vi "Select message creator.vi"(8 "error in (no error)":errorcluster, 11 "Select control references":T2) -> (0 "error out":errorcluster, 3 "PartDetails":T1)   [LabVIEW 2019, in "ZenGage v3.0 UI.lvclass"]
uses:
  ZenGage v3.0 UI.lvclass
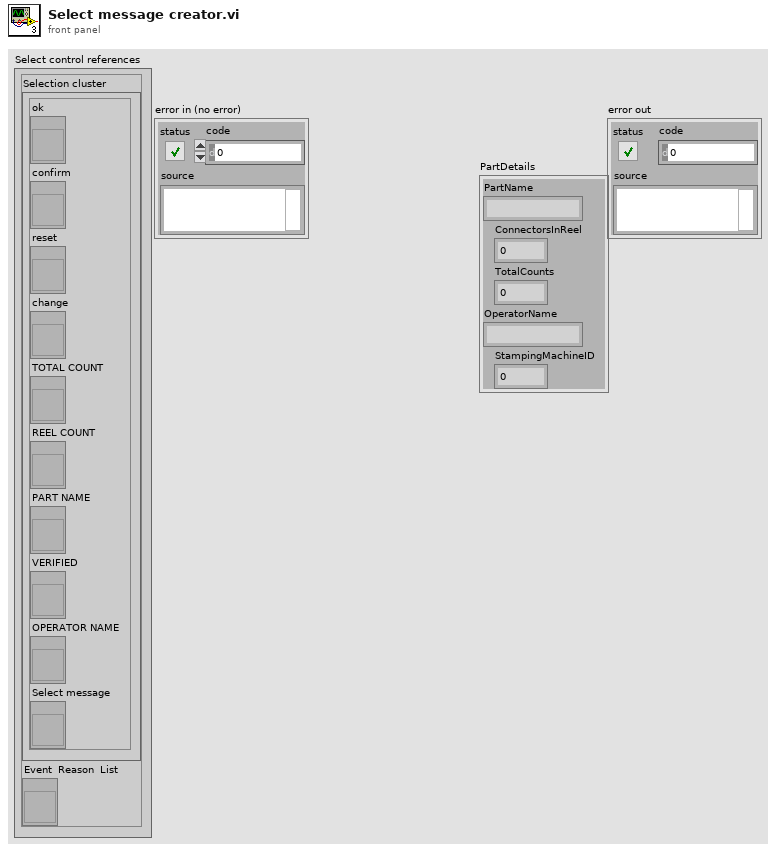
[diagram p1: front panel]
types:
  T1 = cluster{"PartName":string, "ConnectorsInReel":u64, "TotalCounts":u64, "OperatorName":string, "StampingMachineID":u32}
  T2 = cluster{"Selection cluster":cluster{"ok":refnum<vi>, "confirm":refnum<vi>, "reset":refnum<vi>, "change":refnum<vi>, "TOTAL COUNT":refnum<vi>, "REEL COUNT":refnum<vi>, "PART NAME":refnum<vi>, "VERIFIED":refnum<vi>, "OPERATOR NAME":refnum<vi>, "Select message":refnum<vi>}, "Event  Reason  List":refnum<vi>}
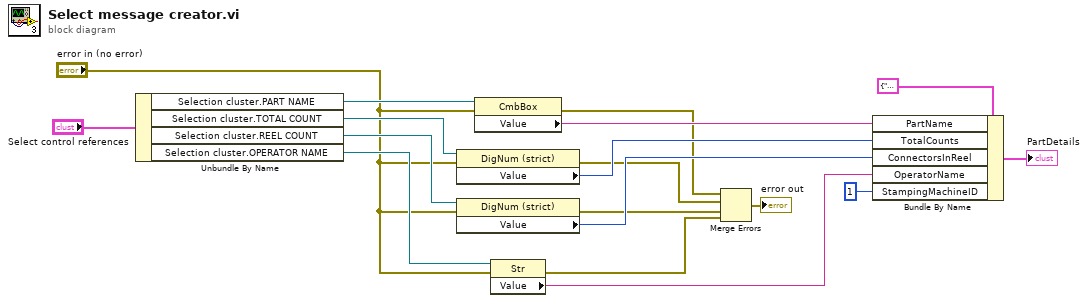
[diagram p0: block diagram]
diagram:
  n1 = Unbundle By Name("Select control references") -> ("Selection cluster.PART NAME"=w17:refnum<vi>, "Selection cluster.TOTAL COUNT"=w16:refnum<vi>, "Selection cluster.REEL COUNT"=w15:refnum<vi>, "Selection cluster.OPERATOR NAME"=w14:refnum<vi>)
  n2 = property class="DigNum (strict)"(reference=w16, error in="error in (no error)") -> (error out=w8:errorcluster, "Value"=w11:u64)  [unwired: 1 out]
  n3 = property class="DigNum (strict)"(reference=w15, error in="error in (no error)") -> (error out=w7:errorcluster, "Value"=w10:u64)  [unwired: 1 out]
  n4 = property class="CmbBox"(reference=w17, error in="error in (no error)") -> (error out=w9:errorcluster, "Value"=w12:string)  [unwired: 1 out]
  n5 = property class="Str"(reference=w14, error in="error in (no error)") -> (error out=w6:errorcluster, "Value"=w2:string)  [unwired: 1 out]
  n6 = Merge Errors(w9, w8, w7, w6) -> (→"error out":errorcluster)
  n7 = Bundle By Name(cluster=T1 {"PartName"="", "ConnectorsInReel"=0, "TotalCounts"=0, "OperatorName"="", "StampingMachineID"=0} ("PartDetails"), "PartName"=w12, "TotalCounts"=w11, "ConnectorsInReel"=w10, "OperatorName"=w2, "StampingMachineID"=u32 1) -> (→"PartDetails":T1)
